vi "Main.vi"() -> ()   [LabVIEW 2018]
doc: "The myRIO Project template acquires acceleration data from the onboard accelerometer and displays the changes of acceleration values in a waveform chart."
uses:
  <vilib>/myRIO/Common/Instrument Driver Framework/myRIO v1.0/UART/vis/myRIO v1.0 Close UART.vi
  <vilib>/myRIO/Common/Instrument Driver Framework/Utilities/vis/FPGA Ref Manager.vi
  <vilib>/myRIO/Common/Instrument Driver Framework/myRIO v1.0/myRIO v1.0 Reset FPGA.vi
  <vilib>/myRIO/Common/Instrument Driver Framework/myRIO v1.0/IRQ/vis/myRIO v1.0 IRQ Info FGV.vi
  <vilib>/myRIO/Common/Instrument Driver Framework/myRIO v1.0/IRQ/vis/myRIO v1.0 Timer IRQ Info FGV.vi
  <vilib>/myRIO/Common/Instrument Driver Framework/myRIO v1.0/IRQ/vis/myRIO v1.0 ISR Agent.vi
  <vilib>/myRIO/Instrument Drivers/Utilities/Utilities.lvlib
panel:
  in  "Kaffee anfordern":bool
  in  "Cluster":cluster{"aktuelle Teperatur":dbl}
  out "error out":errorcluster
  in  "Stop":bool
  # "Overview: The myRIO Project template acquires acceleration data from the onboard accelerometer and displays the changes of acceleration values in a waveform chart.\nInstructions:\n1. Check the myRIO target IP address in the project and make sure the target IP address is correct. \n2. Run this VI."
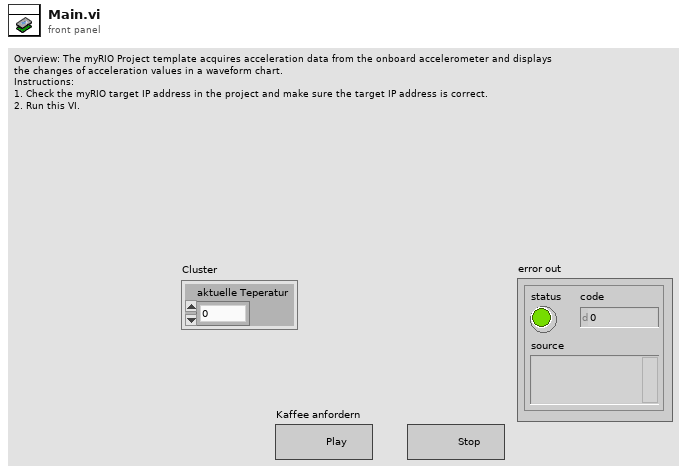
[diagram p1: front panel]
types:
  T1 = enum16{"Idle", "Emergency-Stop", "Pumpen", "Heizen"}
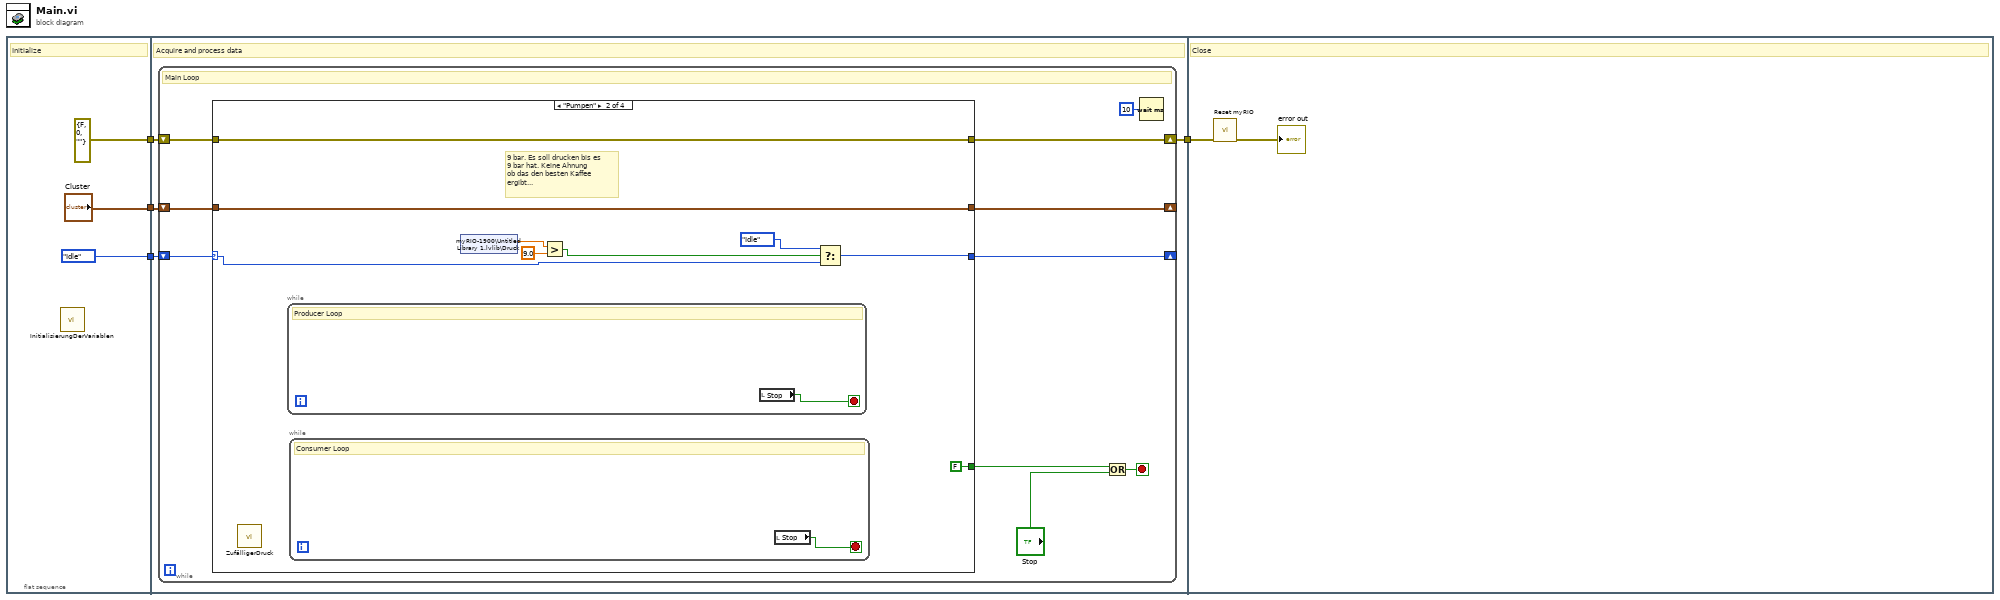
[diagram p0: block diagram]
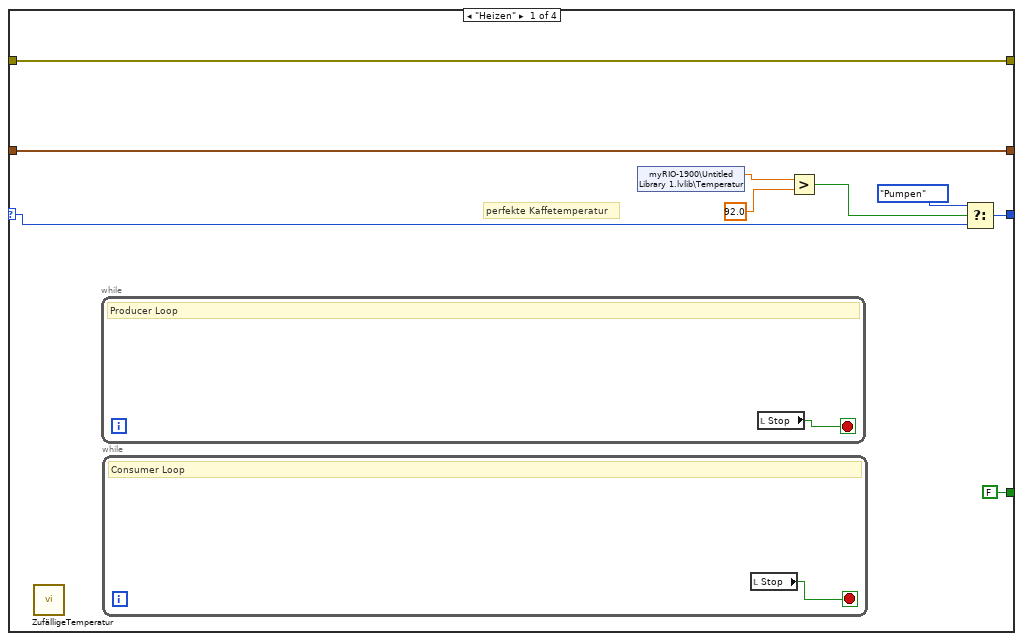
[diagram p2: hidden frame]
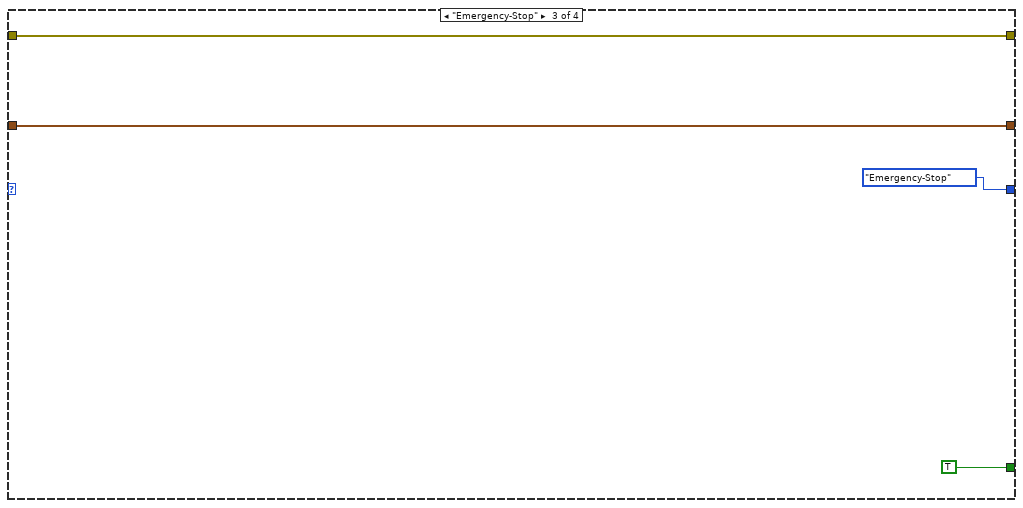
[diagram p3: hidden frame]
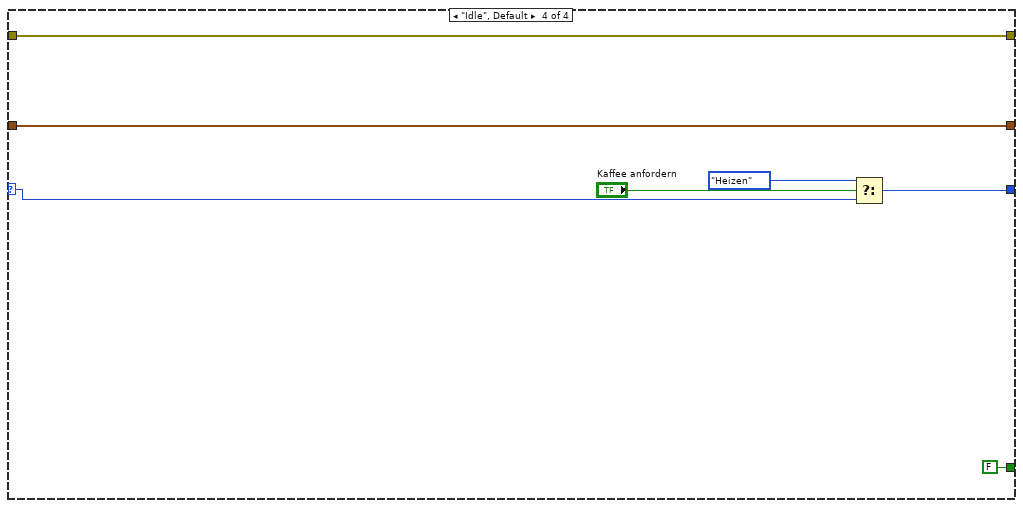
[diagram p4: hidden frame]
diagram:
  n1 = flat-sequence {
    tunnel: [errorcluster {"status"=FALSE, "code"=0, "source"=""} ("error in (no error)")] -> w4
    tunnel: [T1."Idle"] -> w2
    tunnel: ["Cluster"] -> w1
    tunnel: w4 -> [w11]
    tunnel: [w10] -> w3
    tunnel: w2 -> [w9]
    tunnel: w1 -> [w8]
    tunnel: w3 -> [w56]
    frame #0 {
      # "Initialize"
      n2 = call "InitialisierungDerVariablen.vi"() -> ()  [unwired: 12 in]
    }
    frame #1 {
      # "Acquire and process data"
      n3 = while {
        shift-right: [w16] -> w10
        shift-left: w11 -> [w18]
        shift-right: [w12] -> _
        shift-left: w9 -> [w19]
        shift-right: [w15] -> _
        shift-left: w8 -> [w17]
        stop <- w21 stop-if-true
        # "Main Loop"
        n4 = case shown="\"Pumpen\"" w19 {
          selector: w19 -> [w26 w35 _ w51]
          tunnel: w18 -> [w30 w41 w47 w54]
          tunnel: w17 -> [w29 w40 w46 w53]
          tunnel: [w30 w41 w47 w54] -> w16
          tunnel: [w29 w40 w46 w53] -> w15
          tunnel: [FALSE FALSE TRUE FALSE] -> w13
          tunnel: [w27 w33 T1."Emergency-Stop" w50] -> w12
          frame "Heizen" {
            # "perfekte Kaffetemperatur"
            n5 = call "ZufälligeTemperatur.vi"() -> ()  [unwired: 12 in]
            n6 = while {
              stop <- w32 stop-if-true
              # "Producer Loop"
              n7 = local read "Stop"() -> (w32:bool)
            }
            n8 = while {
              stop <- w31 stop-if-true
              # "Consumer Loop"
              n9 = local read "Stop"() -> (w31:bool)
            }
            n10 = shared-variable "myRIO-1900\\Untitled Library 1.lvlib\\Temperatur"() -> (w25:dbl)  [unwired: 1 in, 1 out]
            n11 = Greater?(x=w25, y=92.0) -> (0:w23:bool)
            n12 = Select(t=T1."Pumpen", s=w23, f=w26) -> (s? t:f=w27:T1)
          }
          frame "Pumpen" {
            # "9 bar. Es soll drucken bis es \n9 bar hat. Keine Ahnung\nob das den besten Kaffee\nergibt..."
            n13 = call "ZufälligerDruck.vi"() -> ()  [unwired: 12 in]
            n14 = while {
              stop <- w43 stop-if-true
              # "Producer Loop"
              n15 = local read "Stop"() -> (w43:bool)
            }
            n16 = while {
              stop <- w42 stop-if-true
              # "Consumer Loop"
              n17 = local read "Stop"() -> (w42:bool)
            }
            n18 = shared-variable "myRIO-1900\\Untitled Library 1.lvlib\\Druck"() -> (w38:dbl)  [unwired: 1 in, 1 out]
            n19 = Greater?(x=w38, y=9.0) -> (0:w36:bool)
            n20 = Select(t=T1."Idle", s=w36, f=w35) -> (s? t:f=w33:T1)
          }
          frame "Emergency-Stop" {
          }
          frame "Idle", Default {
            n21 = Select(t=T1."Heizen", s="Kaffee anfordern", f=w51) -> (s? t:f=w50:T1)
          }
        }
        n22 = Or(x=w13, y="Stop") -> (x .or. y?=w21:bool)
        n23 = Wait (ms)(milliseconds to wait=u32 10) -> ()  [unwired: 1 out]
      }
    }
    frame #2 {
      # "Close"
      n24 = call <vilib>:"Reset myRIO.vi"("error in (no error)"=w56) -> ("error out"=→"error out":errorcluster)  [unwired: 10 in]
    }
  }
